vi "Get Iteration and Late Count.vi"(8 "error in (no error)":errorcluster, 11 "Transfer Group in":refnum<class "Transfer Group.lvclass">) -> (0 "error out":errorcluster, 1 "late count":i32, 2 "iteration":u64=1, 3 "Transfer Group out":refnum<class "Transfer Group.lvclass">)   [LabVIEW 2020, in "DSF Core.lvlib" / "Transfer Group.lvclass"]
uses:
  Transfer Group.lvclass
  Transfer Group.lvclass/Transfer Group.ctl
  Timing/Timing.lvclass/Timing.ctl
  Timing/Timing.lvclass
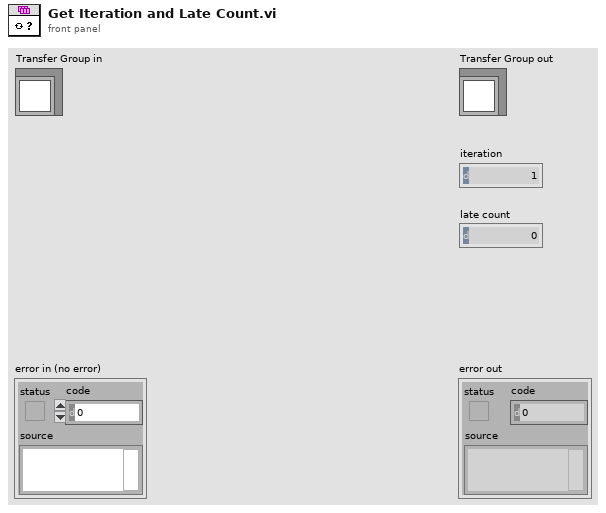
[diagram p1: front panel]
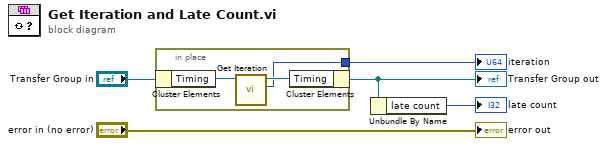
[diagram p0: block diagram]
diagram:
  n1 = in-place {
    in-place-border: [w6] -> w3
    n2 = in-place-cluster #1("Transfer Group in") -> ("Timing"=w8:refnum<class "Timing.lvclass">)
    n3 = call "Get Iteration.vi"("Timing in"=w8) -> ("Iteration"=w6:u64, "Timing out"=w7:refnum<class "Timing.lvclass">)  [unwired: 9 in]
    n4 = in-place-cluster #1("Timing"=w7) -> (w2:refnum<class "Transfer Group.lvclass">)
  }
  "Transfer Group out" <- w2
  "iteration" <- w3
  n5 = Unbundle By Name(w2) -> ("late count"=→"late count":i32)
  "error out" <- "error in (no error)"
